vi "Msg.vi"(7 "Actor in":refnum<class "Actor.lvclass">, 11 "Queue Last Ack Msg in":refnum<class "Queue Last Ack Msg.lvclass">) -> (5 "Actor out":refnum<class "Actor.lvclass">)   [LabVIEW 2021, in "jettl.lvlib" / "Queue Last Ack.lvlib" / "Queue Last Ack Msg.lvclass"]
uses:
  Queue Last Ack Msg.lvclass
  jettl/Actor/Actor.lvclass
  Queue Last Ack/Queue Last Ack.lvclass
  Queue Last Ack Msg.lvclass/Queue Last Ack Msg.ctl
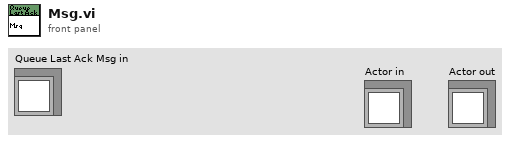
[diagram p1: front panel]
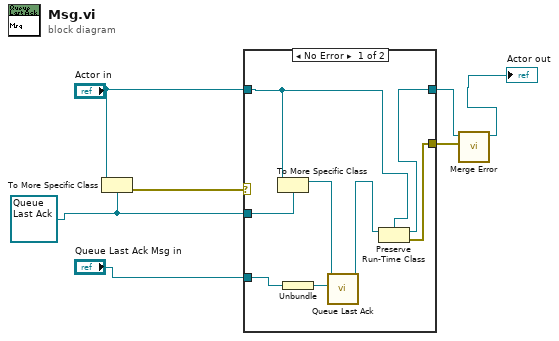
[diagram p0: block diagram]
diagram:
  w5 = refnum<class "Queue Last Ack.lvclass"> refnum ("Last Ack.lvlib:Last Ack.lvclass")
  n1 = To More Specific Class(target class=w5, reference="Actor in") -> (error out=w7:errorcluster)  [unwired: 1 in, 1 out]
  n2 = case shown="No Error" w7 {
    selector: w7 -> [_ w16]
    tunnel: [w9 w17] -> w4
    tunnel: "Actor in" -> [w11 w17]
    tunnel: w5 -> [w15 _]
    tunnel: "Queue Last Ack Msg in" -> [w13 _]
    tunnel: [w8 w16] -> w3
    frame No Error {
      n3 = To More Specific Class(target class=w15, reference=w11) -> (specific class reference=w14:refnum<class "Queue Last Ack.lvclass">)  [unwired: 1 in, 1 out]
      n4 = Unbundle(w13) -> (w12:refnum<class "Queue Actor.lvclass">)
      n5 = call-dynamic "Queue Last Ack.vi"("Queue Actor"=w12, "Queue Last Ack in"=w14) -> ("Queue Last Ack out"=w10:refnum<class "Queue Last Ack.lvclass">)  [unwired: 9 in]
      n6 = Preserve Run-Time Class(object in=w10, 2:w11) -> (object out=w9:refnum<class "Actor.lvclass">, error out=w8:errorcluster)  [unwired: 1 in]
    }
    frame Error {
    }
  }
  n7 = call-dynamic "Merge Error.vi"("Error"=w3, "Set Error in"=w4) -> ("Set Error out"=→"Actor out":refnum<class "Actor.lvclass">)  [unwired: 9 in]
